vi "Raw_input_to_sorted.vi"(10 "Input Array":dbl[](array[numeric])) -> (3 "Array Out":dbl[](array[numeric]))   [LabVIEW 2016]
doc: "This SubVI takes in Raw Serial Data and sorts it according to its adress"
panel:
  in  "New array":dbl[](array[numeric])=[0.0, 0.0, 0.0, 0.0, 0.0, 0.0, 0.0, 0.0, 0.0, 0.0, 0.0, 0.0, 0.0, 0.0, 0.0, 0.0, 0.0, 0.0, 0.0, 0.0, 0.0, 0.0, 0.0, 0.0, 0.0, 0.0, 0.0, 0.0, 0.0, 0.0, 0.0, 0.0, 0.0, 0.0, 0.0, 0.0, 0.0, 0.0, 0.0]
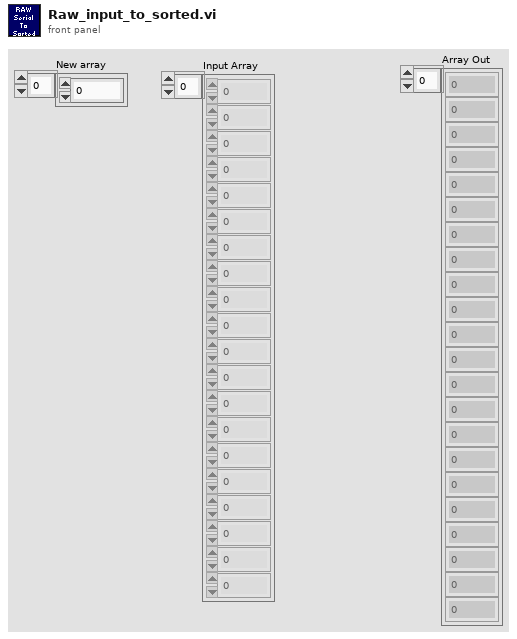
[diagram p1: front panel]
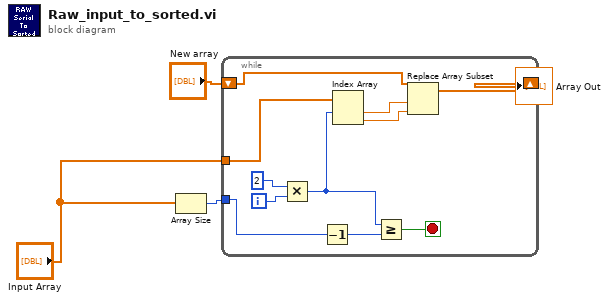
[diagram p0: block diagram]
diagram:
  n1 = Array Size(array="Input Array") -> (size(s)=w2:i32)
  n2 = while {
    tunnel: "Input Array" -> [w15]
    tunnel: w2 -> [w10]
    shift-right: [w5] -> w4
    shift-left: "New array" -> [w6]
    i -> [w12]
    stop <- w7 stop-if-true
    n3 = Multiply(x=2, y=w12) -> (x*y=w8:i32)
    n4 = Decrement(x=w10) -> (x-1=w9:i32)
    n5 = Index Array(array=w15, index #1=w8) -> (element #1=w14:dbl, element #2=w13:dbl)  [unwired: 1 in]
    n6 = Greater Or Equal?(x=w8, y=w9) -> (x >= y?=w7:bool)
    n7 = Replace Array Subset(array=w6, new element=w13, index=w14) -> (w5:dbl[])
  }
  "Array Out" <- w4
